vi "About.vi"(8 "error in":errorcluster, 11 "Timeout (ms)":i32=1000) -> (0 "error out":errorcluster)   [LabVIEW 2018]
doc: "Display the application About dialog. This is a modal window.\n\nSelf-closes after specified timeout. Also, a hidden button the size of the entire dialog allows a mouse down event to close the window. Alternately, a mouse down event for the VI/panel could be programmed to close the dialog box.\n\nBe sure to modify window title for each application.\n\nCopyright © 2019 Epimedia, Inc. All Rights Reserved.\n\nThe Epimedia Application Library is Copyright © 2009-2019 Epimedia, Inc. \nAll Rights Reserved. Used under license."
panel:
  in  "Exit":bool
  # "Copyright © 2019 Epimedia, Inc. All Rights Reserved.\n\nThe Epimedia Application Library is Copyright © 2009-2019 Epimedia, Inc. \nAll Rights Reserved. Used under license."
  # "Click Anywhere in this window to Exit"
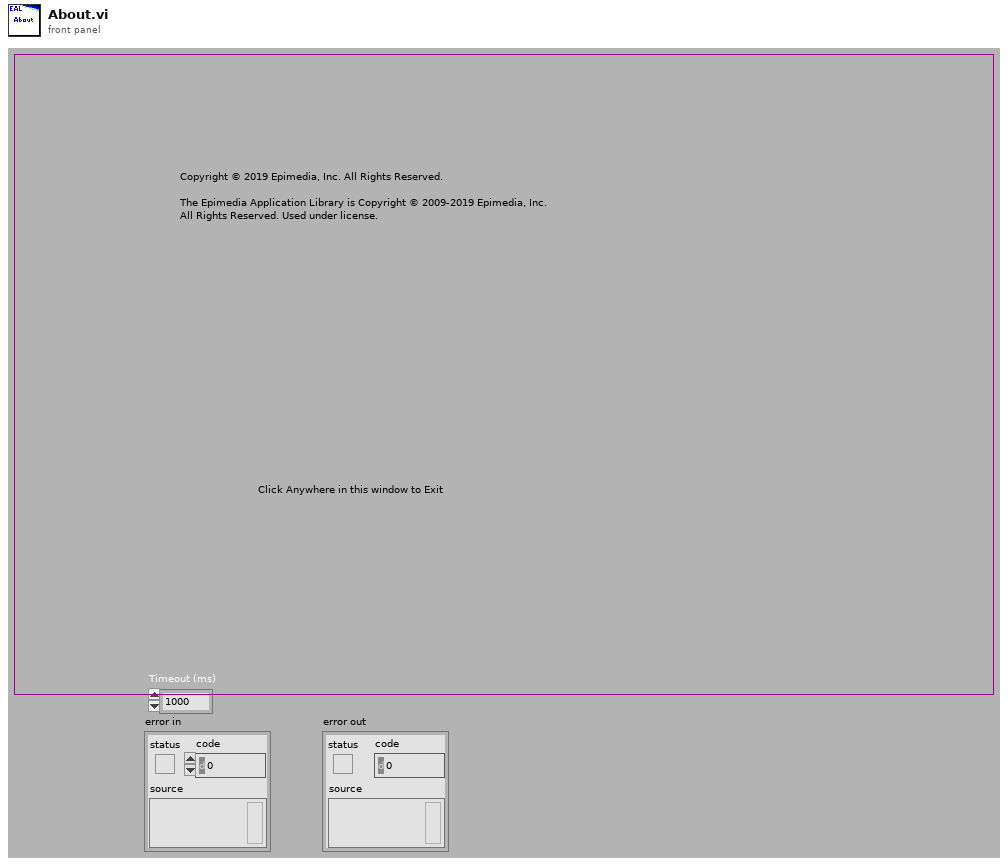
[diagram p1: front panel]
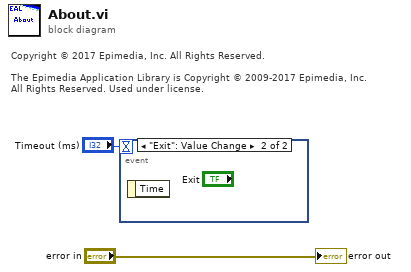
[diagram p0: block diagram]
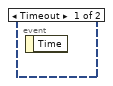
[diagram p2: hidden frame]
diagram:
  # "Copyright © 2017 Epimedia, Inc. All Rights Reserved.\n\nThe Epimedia Application Library is Copyright © 2009-2017 Epimedia, Inc. \nAll Rights Reserved. Used under license."
  n1 = event shown="[1] \"Exit\": Value Change" {
    selector: _ -> [_ _]
    dyn-events: _ -> [_ _]
    timeout: "Timeout (ms)" -> [_ _]
    event Timeout {
      n2 = event-data() -> ()  [unwired: 2 out]
    }
    event "Exit": Value Change {
      n3 = event-data() -> ()  [unwired: 2 out]
    }
  }
  "error out" <- "error in"
